vi "Dispatch Tx.vi"(8 "error in (no error)":errorcluster, 10 "framework iteration":u64, 11 "Dispatcher in":refnum<class "Dispatcher.lvclass">) -> (0 "error out":errorcluster, 3 "Dispatcher out":refnum<class "Dispatcher.lvclass">)   [LabVIEW 2017, in "DSF Core.lvlib" / "Dispatcher.lvclass"]
uses:
  Dispatcher.lvclass
  Dispatcher.lvclass/Dispatcher.ctl
  Plugin/Plugin.lvclass/Plugin.ctl
  Timing/Timing.lvclass/Timing.ctl
  Plugin/Get Timing.vi
  Timing/Is Active Cycle.vi
  Timing/Get Decimation.vi
  Timing/Get Offset.vi
  Plugin/Plugin.lvclass
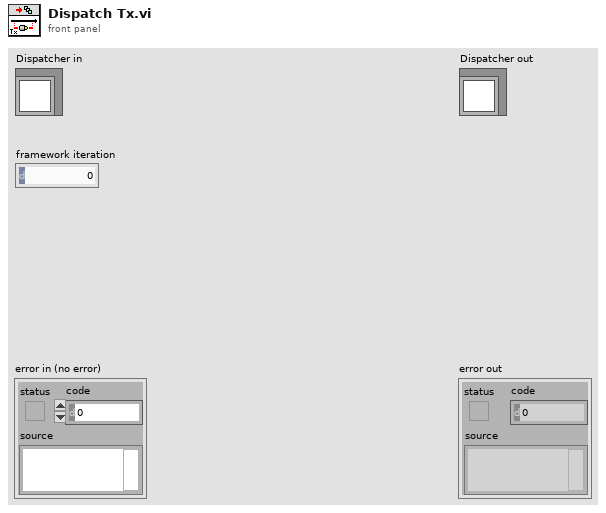
[diagram p1: front panel]
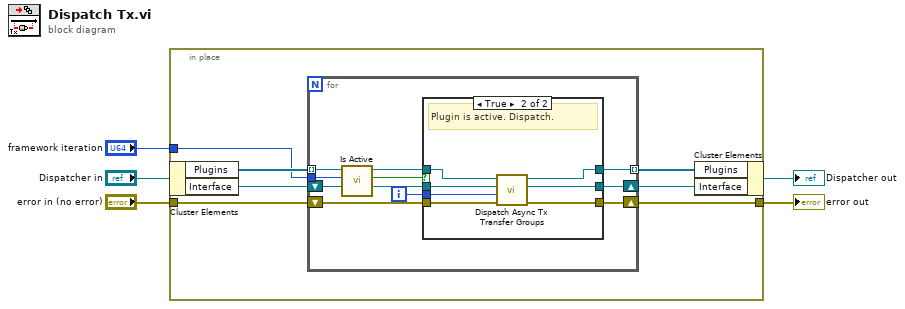
[diagram p0: block diagram]
diagram:
  n1 = in-place {
    in-place-border: "framework iteration" -> [w6]
    in-place-border: "error in (no error)" -> [w12]
    in-place-border: [w11] -> w3
    n2 = in-place-cluster #1("Dispatcher in") -> ("Plugins"=w10:refnum<class "Plugin.lvclass">[], "Interface"=w8:refnum<class "Dispatcher Interface.lvclass">)
    n3 = for {
      tunnel: w10 -> [w19] mode=indexing
      shift-right: [w22] -> w11
      shift-left: w12 -> [w21]
      tunnel: w6 -> [w20]
      tunnel: [w15] -> w9 mode=indexing
      shift-right: [w13] -> w7
      shift-left: w8 -> [w14]
      i -> [w17]
      n4 = call "Is Active.vi"("cycle count"=w20, "Plugin in"=w19) -> ("active this cycle?"=w18:bool, "Plugin out"=w16:refnum<class "Plugin.lvclass">)  [unwired: 8 in]
      n5 = case shown="True" w18 {
        tunnel: [w25 w31] -> w22
        tunnel: w21 -> [w25 w32]
        tunnel: w17 -> [_ w30]
        tunnel: w16 -> [w23 w29]
        tunnel: [w23 w28] -> w15
        tunnel: w14 -> [w24 w27]
        tunnel: [w24 w26] -> w13
        frame False {
          # "Plugin is not active. Skip."
        }
        frame True {
          # "Plugin is active. Dispatch."
          n6 = call "Dispatch Async Tx Transfer Groups.vi"("error in (no error)"=w32, "Plugin ID"=w30, "Dispatcher Interface in"=w27, "Plugin in"=w29) -> ("error out"=w31:errorcluster, "Dispatcher Interface out"=w26:refnum<class "Dispatcher Interface.lvclass">, "Plugin out"=w28:refnum<class "Plugin.lvclass">)  [unwired: 5 in]
        }
      }
    }
    n7 = in-place-cluster #1("Plugins"=w9, "Interface"=w7) -> (→"Dispatcher out":refnum<class "Dispatcher.lvclass">)
  }
  "error out" <- w3
